vi "Main.vi"(7 "Action":T1=enum."Close", 8 "Error In":errorcluster, 11 "File Path to Load":path) -> (0 "Error Out":errorcluster, 3 "Output":variant)   [LabVIEW 2018, in "Image Management.lvlib"]
doc: "Action Engine for the module. This private VI is wrapped for the API."
uses:
  Image Management.lvlib
  Action.ctl
  <vilib>/vision/Image Controls.llb/IMAQ Image.ctl
  <vilib>/Utility/error.llb/Error Cluster From Error Code.vi
  <vilib>/ErrorRing/Error Ring.xnode
panel:
  in  "Data in (not used...yet)":variant
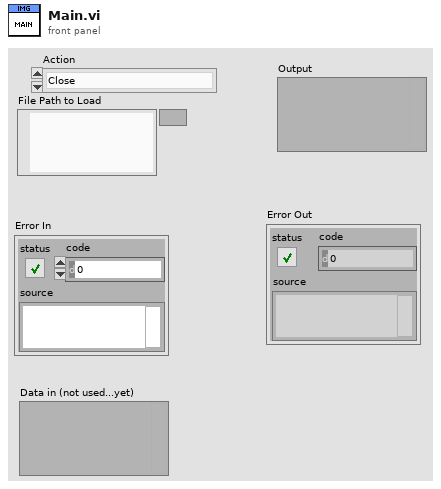
[diagram p1: front panel]
types:
  T1 = typedef "Image Management.lvlib/Action.ctl" = enum16{"Init", "Open Image in Default Program", "Find Linespaces", "Get Image Size (pixels)", "Close"}
  T2 = typedef "IMAQ Image.ctl" = refnum<image>
  T3 = cluster{"File Path":path, "Image Pixels (U8)":u8[][], "Rows where whitespace starts":i32[], "Receipt Image Ref":T2}
  T4 = cluster{"Image Pixels (U8)":u8[][], "Image Out":T2}
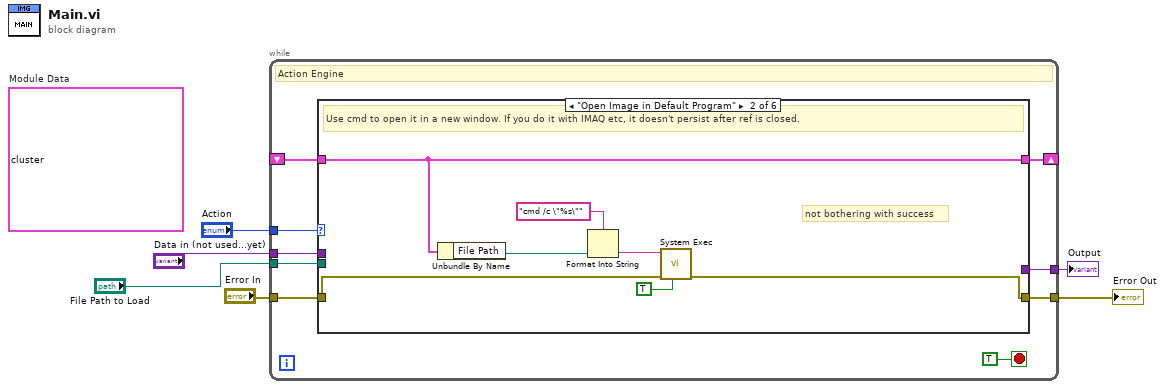
[diagram p0: block diagram]
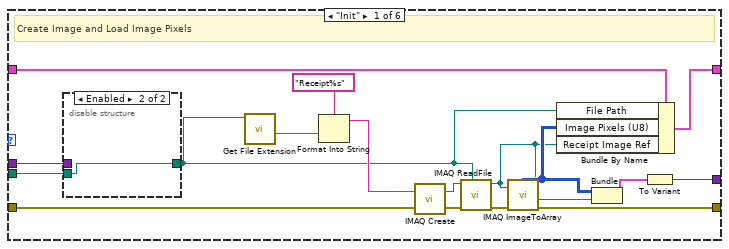
[diagram p2: hidden frame]
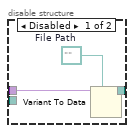
[diagram p3: hidden frame]
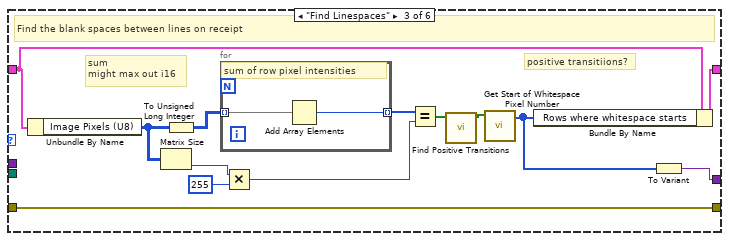
[diagram p4: hidden frame]
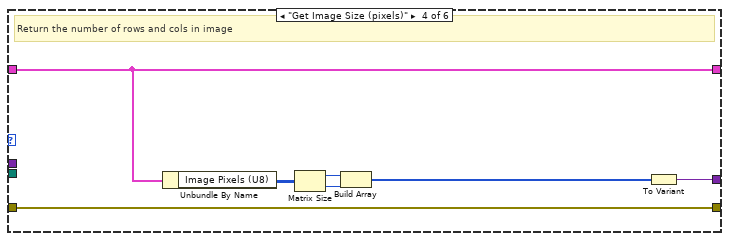
[diagram p5: hidden frame]
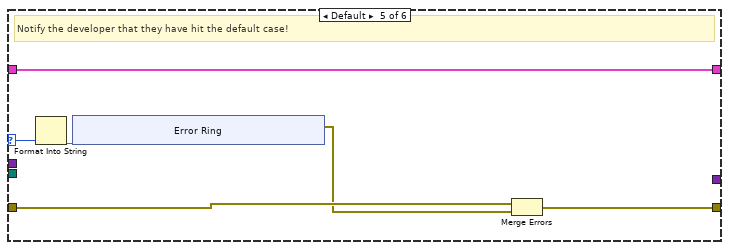
[diagram p6: hidden frame]
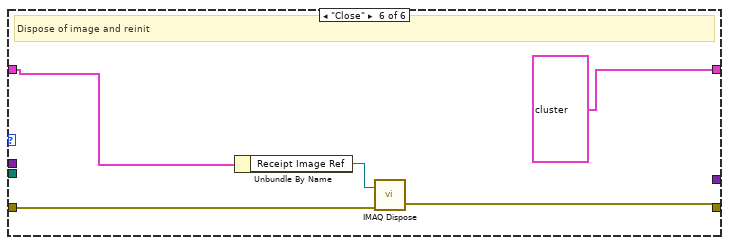
[diagram p7: hidden frame]
diagram:
  (unwired) T3 {"File Path"=path "", "Image Pixels (U8)"=[], "Rows where whitespace starts"=[], "Receipt Image Ref"=refnum}  # Module Data
  n1 = while {
    tunnel: "Error In" -> [w13]
    tunnel: [w14] -> w5
    tunnel: "Action" -> [w12]
    shift-right: [w11] -> _
    shift-left: _ -> [w10]
    tunnel: "Data in (not used...yet)" -> [w9]
    tunnel: "File Path to Load" -> [w8]
    tunnel: [w7] -> w1
    stop <- TRUE stop-if-true
    # "Action Engine"
    n2 = case shown="\"Open Image in Default Program\"" w12 {
      selector: w12 -> [_ _ _ _ w67 _]
      tunnel: [w29 w38 w46 w64 w71 w82] -> w14
      tunnel: w13 -> [w30 w39 w46 w64 w70 w83]
      tunnel: [w22 w42 w47 w59 w66 T3 {"File Path"=path "", "Image Pixels (U8)"=[], "Rows where whitespace starts"=[], "Receipt Image Ref"=refnum}] -> w11
      tunnel: w10 -> [w25 w42 w48 w59 w66 w81]
      tunnel: w9 -> [w24 _ _ _ _ _]
      tunnel: w8 -> [w21 _ _ _ _ _]
      tunnel: [w20 _ w44 w63 _ _] -> w7
      frame "Init" {
        # "Create Image and Load Image Pixels"
        n3 = disable-structure shown="Enabled" {
          disable-tunnel: w24 -> [w35 _]
          disable-tunnel: [w33 w36] -> w19
          disable-tunnel: w21 -> [_ w36]
          frame Disabled {
            w34 = path ""  # File Path
            n4 = Variant To Data(type=w34, Variant=w35) -> (data=w33:path)  [unwired: 1 in, 1 out]
          }
          frame Enabled {
          }
        }
        n5 = call <vilib>:"Get File Extension.vi"("file"=w19) -> ("filename without extension"=w26:string)  [unwired: 6 in, 4 out]
        n6 = Format Into String(format string="Receipt%s" ("Image Name"), w26) -> (resulting string=w23:string)  [unwired: 2 in, 1 out]
        n7 = call "IMAQ Create"("Image Name"=w23, "error in (no error)"=w30) -> ("New Image"=w32:T2, "error out"=w31:errorcluster)  [unwired: 3 in]
        n8 = call "IMAQ ReadFile"("File Path"=w19, "error in (no error)"=w31, "Image"=w32) -> ("error out"=w28:errorcluster, "Image Out"=w17:T2)  [unwired: 4 in, 3 out]
        n9 = call "IMAQ ImageToArray"("error in (no error)"=w28, "Image"=w17) -> ("error out"=w29:errorcluster, "Image Pixels (U8)"=w18:u8[][])  [unwired: 2 in, 3 out]
        n10 = Bundle By Name(cluster=w25, "File Path"=w19, "Image Pixels (U8)"=w18, "Receipt Image Ref"=w17) -> (w22:T3)
        n11 = Bundle("Image Pixels (U8)"=w18, "Image Out"=w17) -> (w16:T4)  [unwired: 1 in]
        n12 = To Variant(anything=w16) -> (Variant=w20:variant)
      }
      frame "Open Image in Default Program" {
        # "not bothering with success"
        # "Use cmd to open it in a new window. If you do it with IMAQ etc, it doesn't persist after ref is closed."
        n13 = Unbundle By Name(w42) -> ("File Path"=w41:path)
        n14 = Format Into String(format string="cmd /c \"%s\"" ("command line"), w41) -> (resulting string=w40:string)  [unwired: 2 in, 1 out]
        n15 = call <vilib>:"System Exec.vi"("run minimized? (F)"=TRUE, "error in (no error)"=w39, "command line"=w40) -> ("error out"=w38:errorcluster)  [unwired: 5 in, 3 out]
      }
      frame "Find Linespaces" {
        # "positive transitiions?"
        # "sum\nmight max out i16"
        # "Find the blank spaces between lines on receipt"
        n16 = Unbundle By Name(w48) -> ("Image Pixels (U8)"=w55:u8[][])
        n17 = Matrix Size(0:w55) -> (2:w54:i32)  [unwired: 1 out]
        n18 = To Unsigned Long Integer(number=w55) -> (unsigned 32bit integer=w56:u32[][])
        n19 = for {
          tunnel: [w58] -> w52 mode=indexing
          tunnel: w56 -> [w57] mode=indexing
          # "sum of row pixel intensities"
          n20 = Add Array Elements(numeric array=w57) -> (sum=w58:u32)
        }
        n21 = Multiply(x=w54, y=255) -> (x*y=w51:i32)
        n22 = Equal?(x=w52, y=w51) -> (x = y?=w50:bool[])
        n23 = call "Find Positive Transitions.vi"("Boolean Array in"=w50) -> ("Positive Transitions"=w49:bool[])  [unwired: 10 in]
        n24 = call "Get Start of Whitespace Pixel Number.vi"("Positive Transitions"=w49) -> ("Row/Col where whitespace starts"=w45:i32[])  [unwired: 10 in]
        n25 = Bundle By Name(cluster=w48, "Rows where whitespace starts"=w45) -> (w47:T3)
        n26 = To Variant(anything=w45) -> (Variant=w44:variant)
      }
      frame "Get Image Size (pixels)" {
        # "Return the number of rows and cols in image"
        n27 = Unbundle By Name(w59) -> ("Image Pixels (U8)"=w65:u8[][])
        n28 = Matrix Size(0:w65) -> (1:w61:i32, 2:w60:i32)
        n29 = Build Array(w61, w60) -> (w62:i32[])
        n30 = To Variant(anything=w62) -> (Variant=w63:variant)
      }
      frame Default {
        # "Notify the developer that they have hit the default case!"
        n31 = Format Into String(w67) -> (resulting string=w68:string)  [unwired: 3 in, 1 out]
        n32 = xnode "Error Ring"("parameter 0"=w68) -> ("error out"=w69:errorcluster)
        n33 = Merge Errors(w70, w69) -> (w71:errorcluster)
      }
      frame "Close" {
        # "Dispose of image and reinit"
        n34 = Unbundle By Name(w81) -> ("Receipt Image Ref"=w80:T2)
        n35 = call "IMAQ Dispose"("Image"=w80, "error in (no error)"=w83) -> ("error out"=w82:errorcluster)  [unwired: 4 in]
      }
    }
  }
  "Error Out" <- w5
  "Output" <- w1
